vi "Exp no 4d Full Subtractor.vi"() -> ()   [LabVIEW 2010]
panel:
  out "BORROW":bool
  out "DIFFERENCE":bool
  in  "C":bool
  in  "B":bool
  in  "A":bool
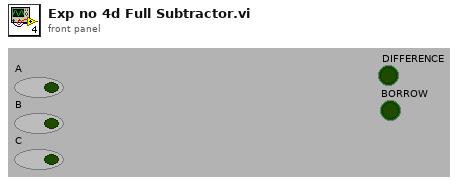
[diagram p1: front panel]
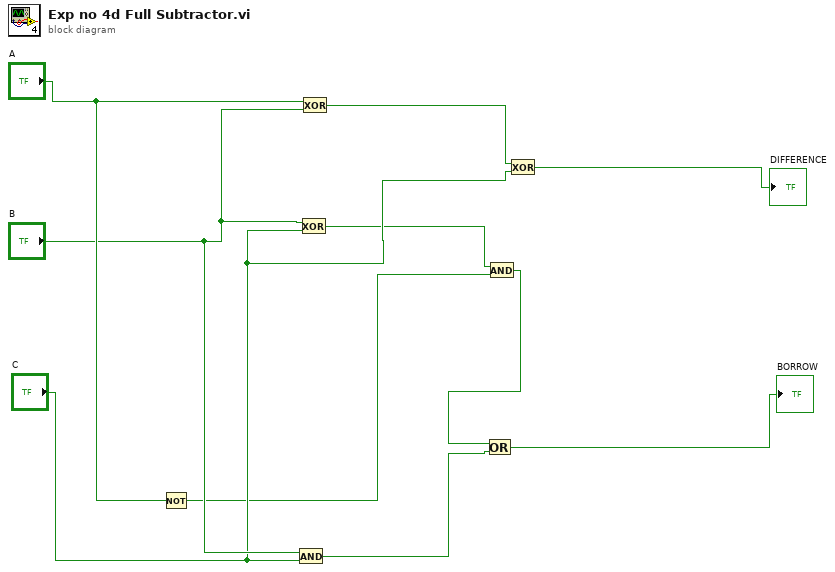
[diagram p0: block diagram]
diagram:
  n1 = Not(x="A") -> (.not. x?=w5:bool)
  n2 = And(x="B", y="C") -> (x .and. y?=w3:bool)
  n3 = Exclusive Or(1:"C", 2:"B") -> (0:w6:bool)
  n4 = Exclusive Or(1:"B", 2:"A") -> (0:w8:bool)
  n5 = And(x=w6, y=w5) -> (x .and. y?=w4:bool)
  n6 = Or(x=w4, y=w3) -> (x .or. y?=→"BORROW":bool)
  n7 = Exclusive Or(1:"C", 2:w8) -> (0:→"DIFFERENCE":bool)
